vi "Digital Input Read Example.vi"() -> ()   [LabVIEW 2020]
uses:
  g_industrial_cam/Camera/Camera.lvclass/Camera.ctl
  g_industrial_cam/Camera/Set Value (String).vi
  g_industrial_cam/Camera/Get Value (Boolean).vi
  g_industrial_cam/Camera/GetSetTrigger.vi
  g_industrial_cam/Camera/GetSetStringValue.vi
  g_industrial_cam/Camera/GetSetBooleanValue.vi
  g_industrial_cam/Camera/Check Not Disconnected.vi
  <vilib>/Utility/error.llb/Error Cluster From Error Code.vi
  g_industrial_cam/Camera/Camera.lvclass
panel:
  in  "stop":bool
  out "Trigger Source Read Loop":i32
  out "Trigger Source Value":bool
  out "Current Trigger Source":string
  out "error out":errorcluster
  out "Trigger Sources":string[](array[string])
  # "This Example Lets You Read the Digital Level on a Physical Trigger Line"
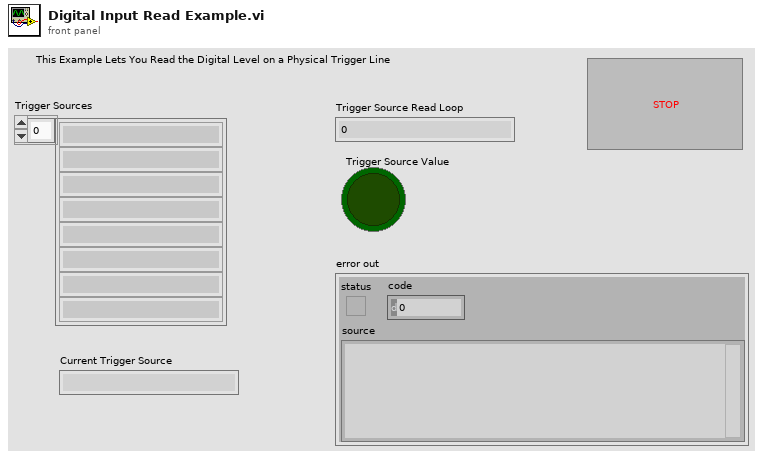
[diagram p1: front panel]
types:
  T1 = typedef "Device Enumeration.ctl" = cluster{"ID":string, "Protocol":string, "Vendor":string, "Model":string, "Serial":string, "Address":string}
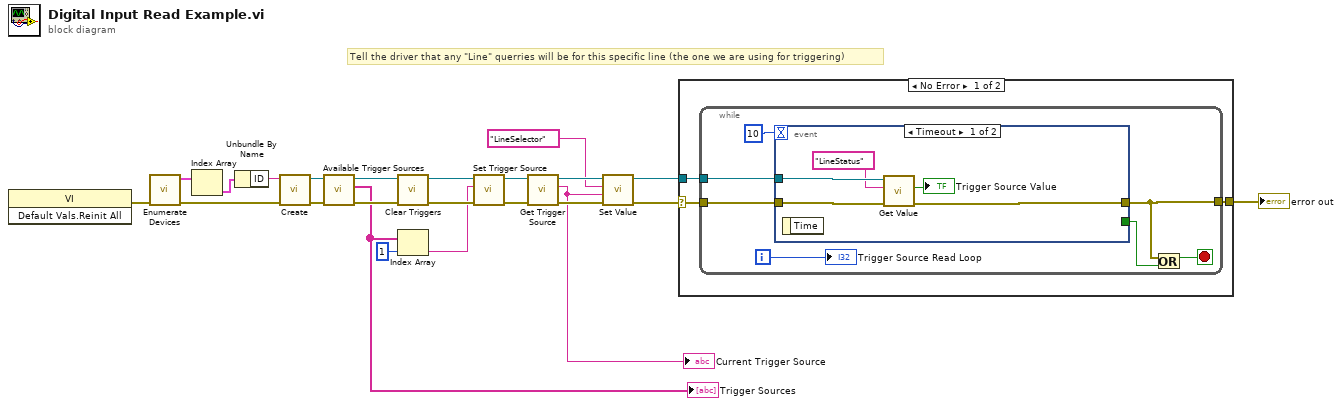
[diagram p0: block diagram]
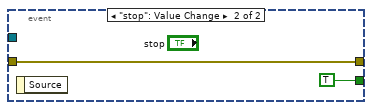
[diagram p2: hidden frame]
diagram:
  # "Tell the driver that any \"Line\" querries will be for this specific line (the one we are using for triggering)"
  n1 = invoke class="VI" method="Default Vals.Reinit All"() -> (error out=w12:errorcluster)  [unwired: 3 in, 2 out]
  n2 = call "Enumerate Devices.vi"("error in (no error)"=w12) -> ("error out"=w22:errorcluster, "Devices"=w23:T1[])  [unwired: 9 in]
  n3 = Index Array(array=w23) -> (element=w21:T1)  [unwired: 1 in]
  n4 = Unbundle By Name(w21) -> ("ID"=w20:string)
  n5 = call "Create.vi"("error in (no error)"=w22, "Identifier (ID, IP etc)"=w20) -> ("error out"=w5:errorcluster, "Camera"=w6:refnum<class "Camera.lvclass">)  [unwired: 8 in]
  n6 = call "Available Trigger Sources.vi"("error in (no error)"=w5, "Camera in"=w6) -> ("error out"=w4:errorcluster, "Available Trigger Sources"=w2:string[], "Camera"=w3:refnum<class "Camera.lvclass">)  [unwired: 7 in]
  "Trigger Sources" <- w2
  n7 = call "Clear Triggers.vi"("error in (no error)"=w4, "Camera in"=w3) -> ("error out"=w9:errorcluster, "Camera"=w8:refnum<class "Camera.lvclass">)  [unwired: 8 in]
  n8 = Index Array(array=w2, index=1) -> (element=w7:string)
  n9 = call "Set Trigger Source.vi"("error in (no error)"=w9, "Source"=w7, "Camera in"=w8) -> ("error out"=w11:errorcluster, "Camera"=w10:refnum<class "Camera.lvclass">)  [unwired: 7 in]
  n10 = call "Get Trigger Source.vi"("error in (no error)"=w11, "Camera in"=w10) -> ("error out"=w19:errorcluster, "Trigger Source"=w13:string, "Camera"=w16:refnum<class "Camera.lvclass">)  [unwired: 7 in]
  "Current Trigger Source" <- w13
  n11 = call-poly "Set Value.vi"("error in (no error)"=w19, "Value"=w13, "Name"="LineSelector", "Camera in"=w16) -> ("error out"=w17:errorcluster, "Camera"=w15:refnum<class "Camera.lvclass">)  [unwired: 6 in]
  n12 = case shown="No Error" w17 {
    selector: w17 -> [w25 w41]
    tunnel: w15 -> [w26 _]
    tunnel: [w24 w41] -> w18
    frame No Error {
      n13 = while {
        tunnel: w26 -> [w33]
        tunnel: w25 -> [w31]
        tunnel: [w30] -> w24
        i -> [w29]
        stop <- w28 stop-if-true
        n14 = event shown="[0] Timeout" {
          selector: _ -> [_ _]
          dyn-events: _ -> [_ _]
          timeout: 10 -> [_ _]
          tunnel: w33 -> [w38 _]
          tunnel: [w37 w40] -> w30
          tunnel: w31 -> [w36 w40]
          tunnel: [_ TRUE] -> w27
          event Timeout {
            n15 = event-data() -> ()  [unwired: 1 in, 1 out]
            n16 = call-poly "Get Value.vi"("error in (no error)"=w36, "Name"="LineStatus", "Camera in"=w38) -> ("error out"=w37:errorcluster, "Value"=→"Trigger Source Value":bool)  [unwired: 6 in, 1 out]
          }
          event "stop": Value Change {
            n17 = event-data() -> ()  [unwired: 1 in, 1 out]
          }
        }
        n18 = Or(x=w30, y=w27) -> (x .or. y?=w28:bool)
        "Trigger Source Read Loop" <- w29
      }
    }
    frame Error {
    }
  }
  "error out" <- w18
